vi "Homogenity.vi"(8 "error in (no error)":errorcluster, 10 "Image in":T2(plugin-control), 11 "Intensity Limit":string[][](array[string])) -> (0 "error out":errorcluster, 2 "Image out":T2(plugin-control), 3 "Homogeneity":T1(array[cluster]))   [LabVIEW 2020]
uses:
  <vilib>/vision/NI_Vision_Development_Module.lvlib
panel:
  out "Result":string
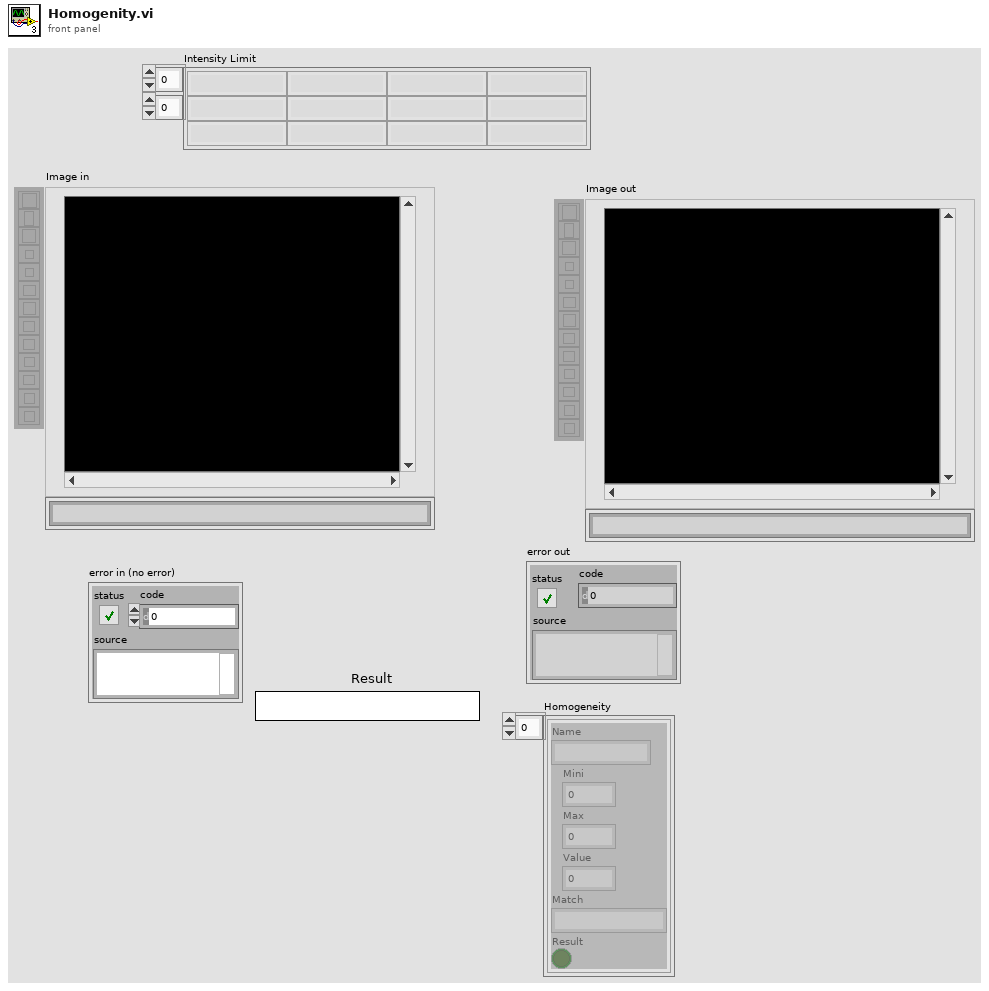
[diagram p1: front panel]
types:
  T1 = cluster{"Name":string, "Mini":dbl, "Max":dbl, "Value ":dbl, "Match":string, "Result":bool}[]
  T2 = typedef "IMAQ Image.ctl" = refnum<image>
  T3 = cluster{"Name":string, "Mini":dbl, "Max":dbl, "Value ":dbl, "Match":string, "Result":bool}
  T4 = cluster{"Global Rectangle":i32[], "Contours":cluster{"Contour Type":u32, "ROI Type":u32, "Points":i32[]}[]}
  T5 = cluster{"Left":i32, "Top":i32, "Right":i32, "Bottom":i32}
  T6 = typedef "IMAQ Rectangle" = cluster{"Left":i32, "Top":i32, "Right":i32, "Bottom":i32, "Rotation":dbl}
  T7 = cluster{"Mean Intensity":sgl, "Standard  Deviation":sgl, "Minimum Intensity":sgl, "Maximum Intensity":sgl}
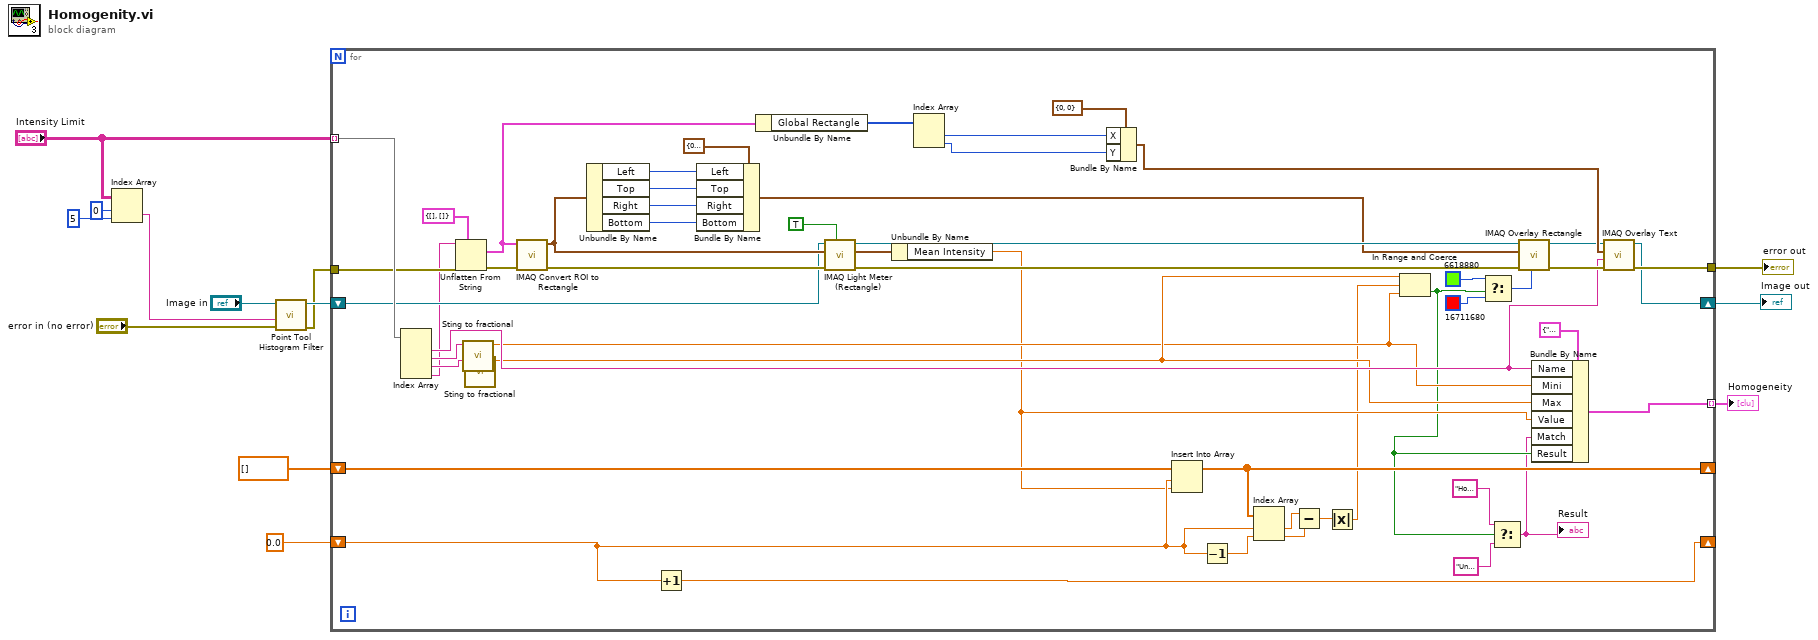
[diagram p0: block diagram]
diagram:
  n1 = Index Array(array="Intensity Limit", index (row)=0, index (col)=5 ("index (row)")) -> (element=w3:string)
  n2 = call "Point Tool Histogram Filter.vi"("error in"="error in (no error)", "Combo Box"=w3, "Image in"="Image in") -> ("error out"=w1:errorcluster, "Image out"=w7:T2)  [unwired: 7 in]
  n3 = for {
    tunnel: "Intensity Limit" -> [w53] mode=indexing
    tunnel: w1 -> [w51]
    shift-right: [w33] -> w12
    shift-left: w7 -> [w50]
    tunnel: [w47] -> w9 mode=indexing
    tunnel: [w42] -> w13
    shift-right: [w28] -> _
    shift-left: dbl[] [] -> [w29]
    shift-right: [w14] -> _
    shift-left: 0.0 -> [w21]
    n4 = Index Array(array=w53) -> (element #1=w32:string, element #2=w49:string, element #3=w48:string, element #4=w31:string)  [unwired: 4 in]
    n5 = Unflatten From String(type=T4 {"Global Rectangle"=[], "Contours"=[]} ("ROI"), binary string=w31, error in (no error)=w51) -> (value=w40:T4, error out=w52:errorcluster)  [unwired: 2 in, 1 out]
    n6 = call "Sting to fractional.vi"("String"=w49) -> ("Numeric"=w20:dbl)  [unwired: 10 in]
    n7 = call "Sting to fractional.vi"("String"=w48) -> ("Numeric"=w30:dbl)  [unwired: 10 in]
    n8 = call "IMAQ Convert ROI to Rectangle"("error in (no error)"=w52, "ROI Descriptor"=w40) -> ("error out"=w55:errorcluster, "Rectangle"=w60:T6)  [unwired: 7 in]
    n9 = Unbundle By Name(w60) -> ("Left"=w59:i32, "Top"=w58:i32, "Right"=w57:i32, "Bottom"=w56:i32)
    n10 = Increment(x=w21) -> (x+1=w14:dbl)
    n11 = Bundle By Name(cluster=T5 {"Left"=0, "Top"=0, "Right"=0, "Bottom"=0} ("Rectangle 2"), "Left"=w59, "Top"=w58, "Right"=w57, "Bottom"=w56) -> (w41:T5)
    n12 = Unbundle By Name(w40) -> ("Global Rectangle"=w39:i32[])
    n13 = call "IMAQ Light Meter (Rectangle)"("Show Search Area"=TRUE, "error in (no error)"=w55, "Rectangle"=w60, "Image"=w50) -> ("error out"=w62:errorcluster, "Gray Level Intensities"=w65:T7, "Image Out"=w63:T2)  [unwired: 3 in, 2 out]
    n14 = Unbundle By Name(w65) -> ("Mean Intensity"=w19:sgl)
    n15 = Index Array(array=w39) -> (element #1=w37:i32, element #2=w36:i32)  [unwired: 2 in]
    n16 = Bundle By Name(cluster=cluster{"X":i32, "Y":i32} {"X"=0, "Y"=0}, "X"=w37, "Y"=w36) -> (w35:cluster{"X":i32, "Y":i32})
    n17 = Insert Into Array "Insert Into Array"(array=w29, index=w21, new element=w19) -> (w28:dbl[])
    n18 = Decrement(x=w21) -> (x-1=w24:dbl)
    n19 = Index Array(array=w28, index #1=w21, index #2=w24) -> (element #1=w23:dbl, element #2=w22:dbl)
    n20 = Subtract(x=w23, y=w22) -> (x-y=w25:dbl)
    n21 = Absolute Value(x=w25) -> (abs(x)=w18:dbl)
    n22 = In Range and Coerce(upper limit=w30, x=w18, lower limit=w20) -> (In Range?=w16:bool)  [unwired: 1 out]
    n23 = Select(t=u32 6618880 ("Color"), s=w16, f=u32 16711680 ("Color")) -> (s? t:f=w44:u32)
    n24 = Select(t="Homogenous", s=w16, f="Un-Homogenous") -> (s? t:f=w15:string)
    "Result" <- w15
    n25 = call "IMAQ Overlay Rectangle"("Color"=w44, "error in (no error)"=w62, "Rectangle"=w41, "Image"=w63) -> ("error out"=w43:errorcluster, "Image Out"=w34:T2)  [unwired: 6 in]
    n26 = Bundle By Name(cluster=T3 {"Name"="", "Mini"=0.0, "Max"=0.0, "Value "=0.0, "Match"="", "Result"=FALSE}, "Name"=w32, "Mini"=w20, "Max"=w30, "Value"=w19, "Match"=w15, "Result"=w16) -> (w47:T3)
    n27 = call "IMAQ Overlay Text"("error in (no error)"=w43, "String"=w32, "Origin"=w35, "Image"=w34) -> ("error out"=w42:errorcluster, "Image Out"=w33:T2)  [unwired: 6 in]
  }
  "Image out" <- w12
  "error out" <- w13
  "Homogeneity" <- w9
